vi "太阳能控制器参数配置.vi"(11 "监测项描述":string) -> ()   [LabVIEW 2016, in "环境动力监测库.lvlib"]
uses:
  <vilib>/Utility/config.llb/NI_LVConfig.lvlib
panel:
  in  "MPPT24低压告警阈值":dbl caption="V"
  in  "MPPT12低压告警阈值":dbl caption="V"
  # "太阳能控制器参数配置"
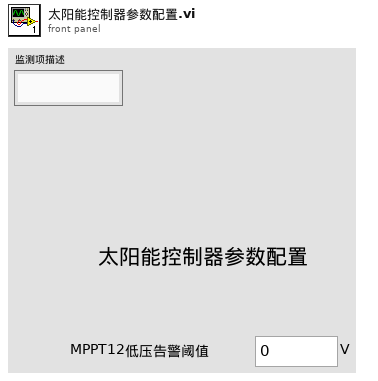
[diagram p1: front panel]
types:
  T1 = typedef "NI_LVConfig.lvlib/Config Data RefNum.ctl" = refnum<k1>
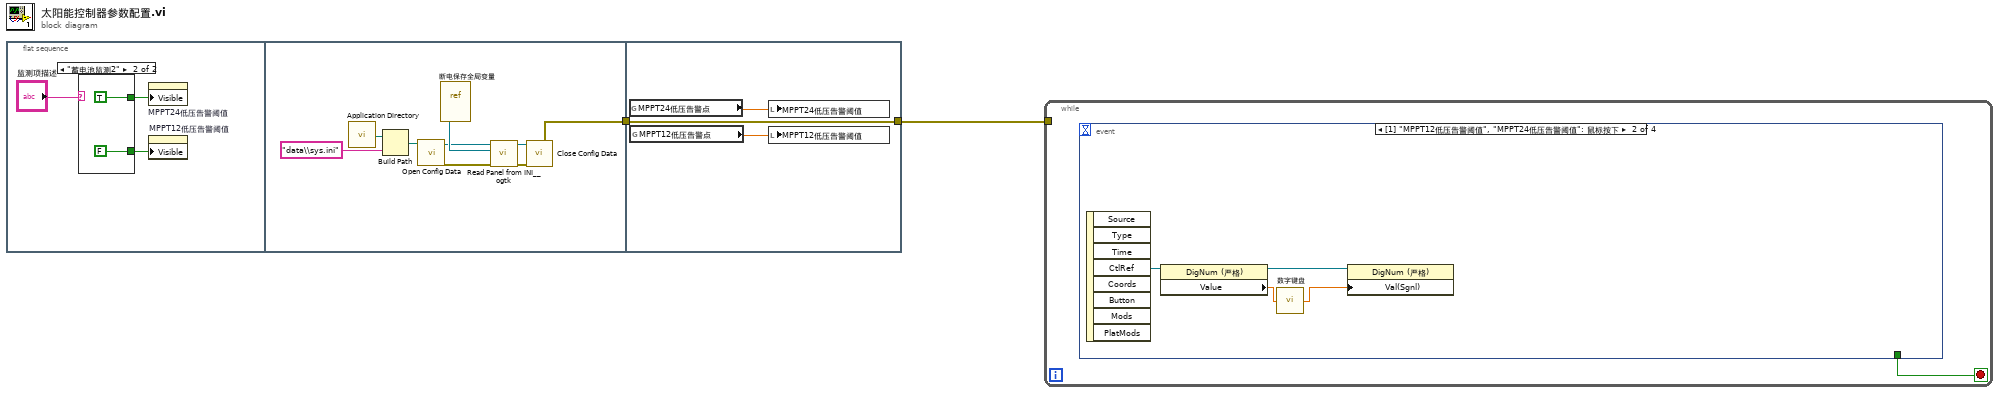
[diagram p0: block diagram]
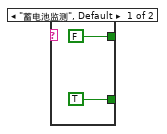
[diagram p2: hidden frame]
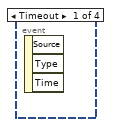
[diagram p3: hidden frame]
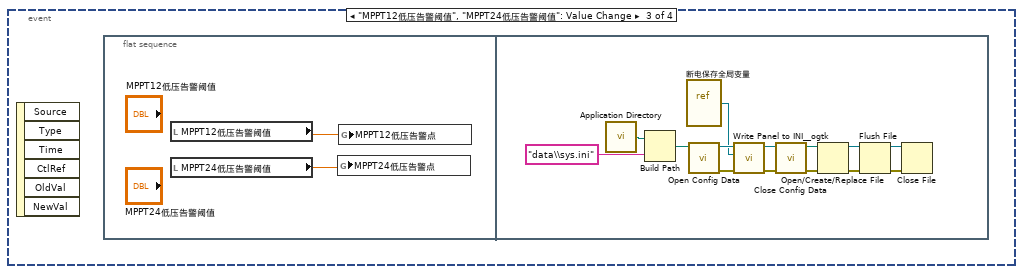
[diagram p4: hidden frame]
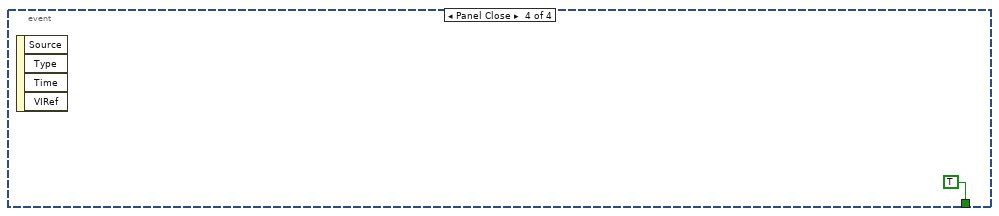
[diagram p5: hidden frame]
diagram:
  n1 = flat-sequence {
    tunnel: [w10] -> w2
    tunnel: [w21] -> w1
    tunnel: w2 -> [w21]
    frame #0 {
      n2 = case shown="\"蓄电池监测2\"" "监测项描述" {
        tunnel: [FALSE TRUE] -> w4
        tunnel: [TRUE FALSE] -> w3
        frame "蓄电池监测", Default {
        }
        frame "蓄电池监测2" {
        }
      }
      n3 = property on="MPPT24低压告警阈值" class="DigNum (严格)"("Visible"=w4) -> ()  [unwired: 2 in, 2 out]
      n4 = property on="MPPT12低压告警阈值" class="DigNum (严格)"("Visible"=w3) -> ()  [unwired: 2 in, 2 out]
    }
    frame #1 {
      n5 = call <vilib>:"Application Directory.vi"() -> ("Application Directory"=w16:path)
      n6 = Build Path(base path=w16, name or relative path="data\\sys.ini" ("名称或相对路径")) -> (appended path=w17:path)
      n7 = call <vilib>:"Open Config Data.vi"("configuration file path"=w17) -> ("error out"=w13:errorcluster, "refnum"=w14:T1)  [unwired: 8 in, 1 out]
      n8 = vi-ref "断电保存全局变量.vi"() -> (w18:refnum<vi>)
      n9 = call <userlib>:"Read Panel from INI__ogtk.vi"("error in (no error)"=w13, "VI ref"=w18, "refnum"=w14) -> ("error out"=w11:errorcluster, "refnum out"=w12:T1)  [unwired: 7 in]
      n10 = call <vilib>:"Close Config Data.vi"("error in (no error)"=w11, "refnum"=w12) -> ("error out"=w10:errorcluster)  [unwired: 8 in, 1 out]
    }
    frame #2 {
      n11 = global read "断电保存全局变量.vi" "MPPT24低压告警点"() -> (w20:dbl)
      n12 = global read "断电保存全局变量.vi" "MPPT12低压告警点"() -> (w19:dbl)
      n13 = local write "MPPT24低压告警阈值"(w20) -> ()
      n14 = local write "MPPT12低压告警阈值"(w19) -> ()
    }
  }
  n15 = while {
    tunnel: w1 -> [_]
    stop <- w22 stop-if-true
    n16 = event shown="[1] \"MPPT12低压告警阈值\", \"MPPT24低压告警阈值\": 鼠标按下" {
      selector: _ -> [_ _ _ _]
      dyn-events: _ -> [_ _ _ _]
      timeout: _ -> [_ _ _ _]
      tunnel: [_ _ _ TRUE] -> w22
      event Timeout {
        n17 = event-data() -> ()  [unwired: 1 in, 3 out]
      }
      event "MPPT12低压告警阈值", "MPPT24低压告警阈值": Mouse Down {
        n18 = event-data() -> ("CtlRef"=w23:refnum<vi>)  [unwired: 1 in, 7 out]
        n19 = property class="DigNum (严格)"(reference=w23) -> (reference out=w25:refnum<vi>, "Value"=w26:dbl)  [unwired: 1 in, 1 out]
        n20 = call "数字键盘.vi"("OldNumber"=w26) -> ("NewNumber"=w24:sgl)
        n21 = property class="DigNum (严格)"(reference=w25, "Val(Sgnl)"=w24) -> ()  [unwired: 1 in, 2 out]
      }
      event "MPPT12低压告警阈值", "MPPT24低压告警阈值": Value Change {
        n22 = event-data() -> ()  [unwired: 1 in, 6 out]
        n23 = flat-sequence {
          frame #0 {
            n24 = local read "MPPT12低压告警阈值"() -> (w28:dbl)
            n25 = local read "MPPT24低压告警阈值"() -> (w27:dbl)
            n26 = global write "断电保存全局变量.vi" "MPPT24低压告警点"(w27) -> ()
            n27 = global write "断电保存全局变量.vi" "MPPT12低压告警点"(w28) -> ()
          }
          frame #1 {
            n28 = call <vilib>:"Application Directory.vi"() -> ("Application Directory"=w42:path)
            n29 = Build Path(base path=w42, name or relative path="data\\sys.ini" ("名称或相对路径")) -> (appended path=w40:path)
            n30 = vi-ref "断电保存全局变量.vi"() -> (w38:refnum<vi>)
            n31 = call <vilib>:"Open Config Data.vi"("configuration file path"=w40) -> ("error out"=w36:errorcluster, "refnum"=w39:T1)  [unwired: 8 in, 1 out]
            n32 = call <userlib>:"Write Panel to INI__ogtk.vi"("error in (no error)"=w36, "VI ref"=w38, "refnum"=w39) -> ("error out"=w35:errorcluster, "refnum out"=w37:T1)  [unwired: 7 in]
            n33 = call <vilib>:"Close Config Data.vi"("error in (no error)"=w35, "refnum"=w37) -> ("error out"=w30:errorcluster, "file path"=w29:path)  [unwired: 8 in]
            n34 = Open/Create/Replace File(file path (use dialog)=w29, error in=w30) -> (refnum out=w33:refnum<file>, error out=w34:errorcluster)  [unwired: 4 in, 1 out]
            n35 = Flush File(refnum=w33, error in=w34) -> (refnum out=w32:refnum<file>, error out=w31:errorcluster)
            n36 = Close File(refnum=w32, error in=w31) -> ()  [unwired: 2 out]
          }
        }
      }
      event Panel Close {
        n37 = event-data() -> ()  [unwired: 1 in, 4 out]
      }
    }
  }
